vi "LeaveDFUSeMode.vi"(0 "Error In":errorcluster, 1 "Max Retries":i32=5, 2 "Working Directory":path=path "") -> (7 "Error":errorcluster, 10 "Success":bool)   [LabVIEW 2010]
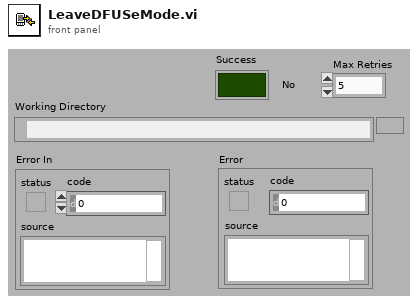
[diagram p1: front panel]
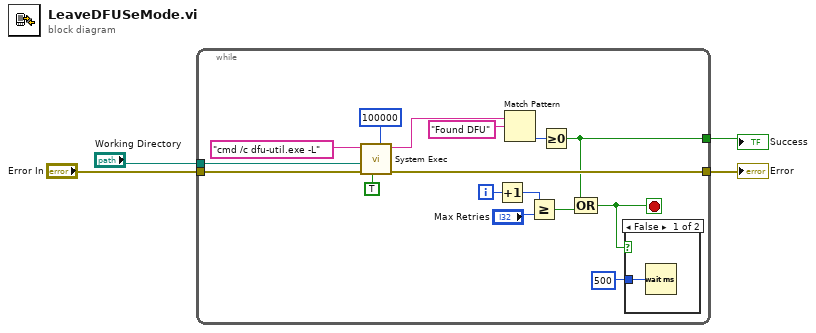
[diagram p0: block diagram]
diagram:
  n1 = while {
    tunnel: "Error In" -> [w20]
    tunnel: "Working Directory" -> [w18]
    tunnel: [w17] -> w3
    tunnel: [w8] -> w2
    i -> [w12]
    stop <- w7 stop-if-true
    n2 = call <vilib>:"System Exec.vi"("expected output size  (4096)"=u32 100000, "run minimized? (F)"=TRUE, "error in (no error)"=w20, "working directory"=w18, "command line"="cmd /c dfu-util.exe -L") -> ("error out"=w17:errorcluster, "standard output"=w15:string)  [unwired: 3 in, 2 out]
    n3 = Increment(x=w12) -> (x+1=w10:i32)
    n4 = Match Pattern(string=w15, regular expression="Found DFU") -> (offset past match=w13:i32)  [unwired: 1 in, 3 out]
    n5 = Greater Or Equal?(x=w10, y="Max Retries") -> (x >= y?=w11:bool)
    n6 = Greater Or Equal To 0?(x=w13) -> (x >= 0?=w8:bool)
    n7 = Compound Arithmetic op=OR(w8, w11) -> (w7:bool)
    n8 = case shown="False" w7 {
      tunnel: u32 500 -> [w21 _]
      frame False {
        n9 = Wait (ms)(milliseconds to wait=w21) -> ()  [unwired: 1 out]
      }
      frame True {
      }
    }
  }
  "Error" <- w3
  "Success" <- w2
